vi "Drive Controller.vi"(8 "error in":errorcluster) -> ()   [LabVIEW 2015]
doc: "This VI executes continuously carrying out the current operation and responding to updates or new operations. It will often contain the timing or control code that is difficult to place directly in TeleOp. This VI generally opens all sensors and motors and isolates the rest of the robot code from knowing how the operations are carried out."
uses:
  Drive Setpoints.ctl
  Drive Operations.ctl
  <vilib>/Rock Robotics/WPI/CAN/TalonSRX/WPI_CANTalonSRX_APIControlMode.ctl
  <vilib>/Rock Robotics/WPI/DriverStation/WPI_DriverStationRobotMode2.ctl
  Drive Published Globals.vi
  Support Code/Team900-VIs/navX Library v2/navX Library v2.lvlib
panel:
  in  "Turn PID Gains (Drive for Distance)":T1 {"derivative time (Td, min)" format="%.3f"; "integral time (Ti, min)" format="%.3f"; "proportional gain (Kc)" format="%.3f"}
  in  "Max Speed":dbl format="%#_13g"
  out "Current\nCmd":string
  # "Tip: It may be helpful to observe inputs and sensor values.\nYou may also want to display tuning or debugging controls."
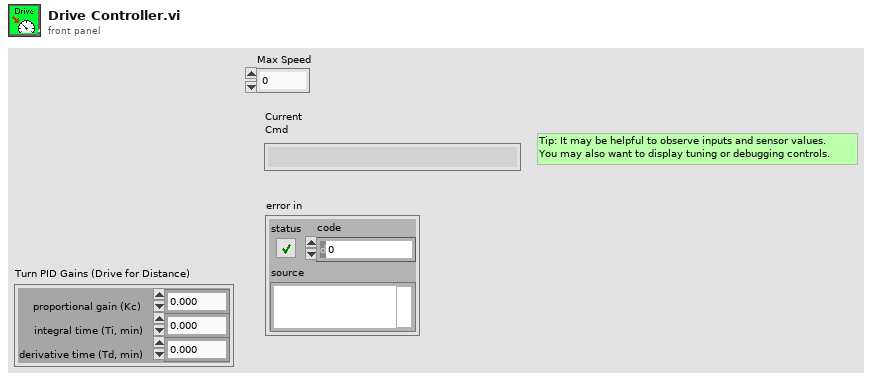
[diagram p1: front panel]
types:
  T1 = cluster{"proportional gain (Kc)":dbl, "integral time (Ti, min)":dbl, "derivative time (Td, min)":dbl}
  T2 = typedef "Drive Setpoints.ctl" = cluster{"Operation":T3, "Left Setpoint":dbl, "Duration":dbl, "Right Setpoint":dbl}
  T3 = typedef "Drive Operations.ctl" = enum16{"Reserve", "Read Current", "Immediate", "Turn to Angle", "Drive for Distance", "Drive for Time"}
  T4 = typedef "Command Status Info.ctl" = cluster{"Name":string, "Status":T5, "notifier out":T6}
  T5 = typedef "Completion Status.ctl" = enum16{"Successful", "Aborted", "Incomplete"}
  T6 = typedef "Completion Notifier.ctl" = refnum<notifier>
  T7 = cluster{"Default Command":T2, "Command Timing":cluster{"Start Time (ms)":u32, "Iterations":i32}, "Command Arguments":cluster{"Command Info":T4, "Description":string, "Default Command":T2, "notifier out":refnum<notifier>, "Subsystem Name":string}}
  T8 = typedef "navX Library v2.lvlib/Z900_navX_DeviceTypeDef.ctl" = cluster{"Interface":cluster{"Protocol":T9, "Update Rate (4Hz-60Hz)":u8, "navX Open TypeDef":variant}, "Notify Packet":refnum<notifier>, "Loop VI Refnum":refnum<vi>, "Ready to Close Occurrence Refnum":refnum<k4>}
  T9 = typedef "navX Library v2.lvlib/Z900_navX_ProtocolTypeDef.ctl" = enum16{"SERIAL", "I2C", "SPI"}
  T10 = typedef "WPI_RobotDriveDevRef.ctl" = cluster{"DevStatus":errorcluster, "Motors[]":T11[], "Square Inputs":bool, "Max Output":dbl}
  T11 = typedef "WPI_MotorControlDeviceRef.ctl" = cluster{"DeviceStatus":errorcluster, "Type":T12, "PWM":cluster{"PWM Channel":T13, "DeadBand":T14}, "CAN":cluster{"Device Number":u8, "Control Mode":T15, "Semaphore":T16, "Max Vout":dbl, "TalonSRX Control Mode":T17}, "Invert":bool}
  T12 = typedef "WPI_MotorControlType.ctl" = enum16{"PWM", "CAN", "CANTalonSRX"}
  T13 = typedef "FPGA_DIOPWMChannel.ctl" = enum8{"PWM 0", "PWM 1", "PWM 2", "PWM 3", "PWM 4", "PWM 5", "PWM 6", "PWM 7", "PWM 8", "PWM 9", "PWM MXP 0", "PWM MXP 1", "PWM MXP 2", "PWM MXP 3", "PWM MXP 4", "PWM MXP 5", "PWM MXP 6", "PWM MXP 7", "PWM MXP 8", "PWM MXP 9", "Invalid"}
  T14 = typedef "WPI_PWMDeadband.ctl" = cluster{"Name":string, "maxPositivePwm":i32, "minPositivePwm":i32, "centerPwm":i32, "maxNegativePwm":i32, "minNegativePwm":i32, "angularRange":u16}
  T15 = typedef "WPI_CANJaguar_ControlMode.ctl" = enum8{"Percent VBus", "Current", "Speed", "Position", "Voltage"}
  T16 = typedef "Semaphore RefNum" = refnum<k1>
  T17 = typedef "WPI_CANTalonSRX_APIControlMode.ctl" = enum8{"Percent VBus", "Speed", "Position", "Slave", "Unchanged / Invalid", "Voltage Compensation", "Current", "Motion Profile"}
  T18 = typedef "WPI_DriverStationRobotMode2.ctl" = enum16{"Autonomous Disabled", "Autonomous Enabled", "Teleop Disabled", "Teleop Enabled", "Disconnected", "Finish", "Test Disabled", "Test Enabled", "Emergency Stopped"}
  T19 = cluster{"Yaw":dbl, "Roll":dbl, "Pitch":dbl, "Heading":dbl, "Fused Heading":dbl}
  T20 = typedef "WPI_CANTalonSRX_GlobalStatus.ctl" = cluster{"Applied Throttle":dbl, "Module Enabled":bool, "CAN Error":errorcluster, "Closed Loop Error":dbl, "Forward Limit Switch Closed":bool, "Reverse Limit Switch Closed":bool, "Sensor Position":dbl, "Sensor Velocity":dbl, "Current":dbl, "Sticky Fault - Over Temp":bool, "Sticky Fault - Under Voltage":bool, "Sticky Fault - Forward Limit":bool, "Sticky Fault - Reverse Limit":bool, "Sticky Fault - Forward Soft Limit":bool, "Sticky Fault - Reverse Soft Limit":bool, "Brake is Enabled":bool, "Encoder Position":dbl, "Encoder Velocity":dbl, "Encoder Index Count":dbl, "Encoder A Pin State":bool, "Encoder B Pin State":bool, "Encoder Index Pin State":bool, "Analog In":dbl, "Analog In Velocity":dbl, "Temperature (C)":dbl, "Battery Voltage":dbl, "Control 5 Is Supported":bool, "Current Profile Slot Select":dbl, "Pos Div 8":bool, "Vel Div 4":bool, "Pulse Width Position":i32, "Pulse Width Velocity":i32, "Pulse Width Rise To Rise (us)":i32, "Pulse Width Rise To Fall (us)":i32, "Mot Prof Active Is Under Run":bool, "Mot Prof Active Has Under Run":bool, "Mot Prof Active Is Last":bool, "Mot Prof Active Velocity Only":bool, "Mot Prof Active Is Valid":bool, "Mot Prof Buffer Is Full":bool, "Mot Prof Active Profile Slot Select":i32, "Mot Prof NextID":i32, "Mot Prof Count":i32, "Mot Prof Active Velocity":dbl, "Mot Prof Active Position":dbl, "Mot Prof Output Enable":i32}
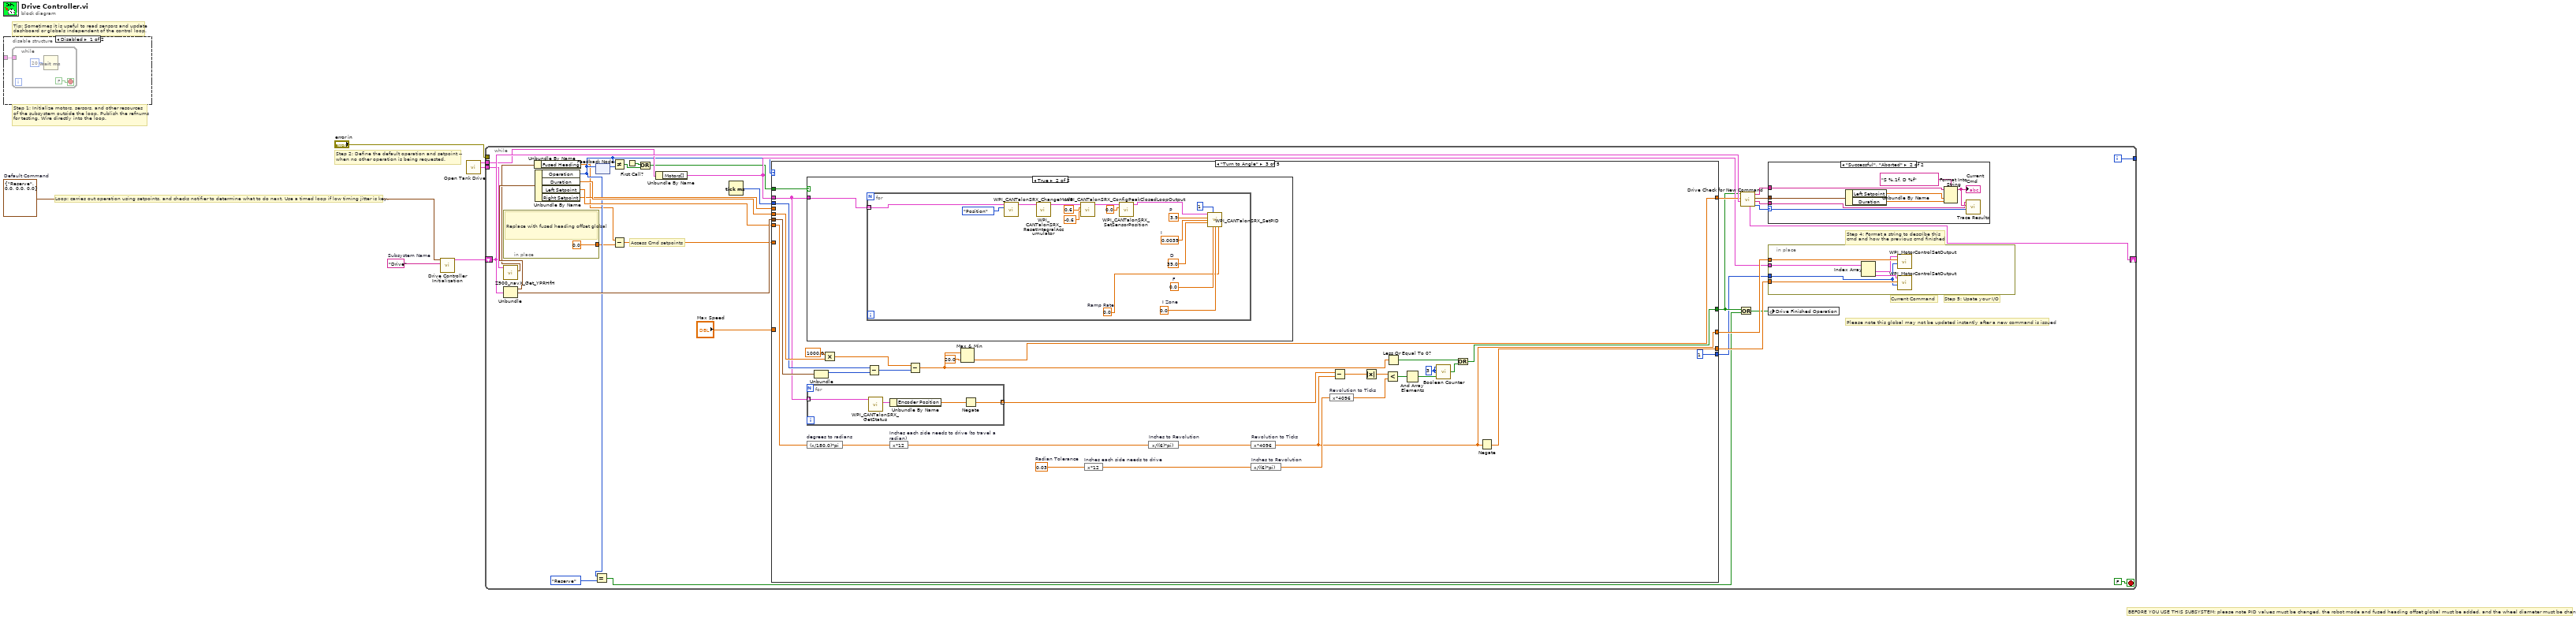
[diagram p0: block diagram]
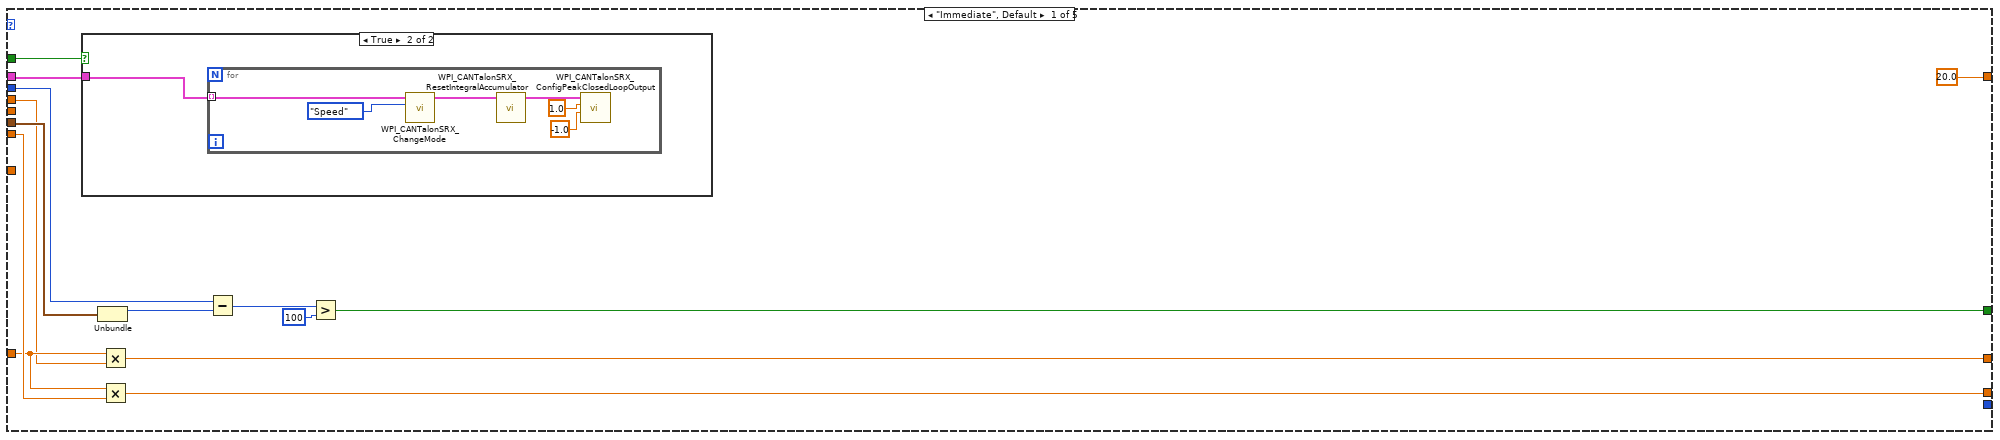
[diagram p4: hidden frame]
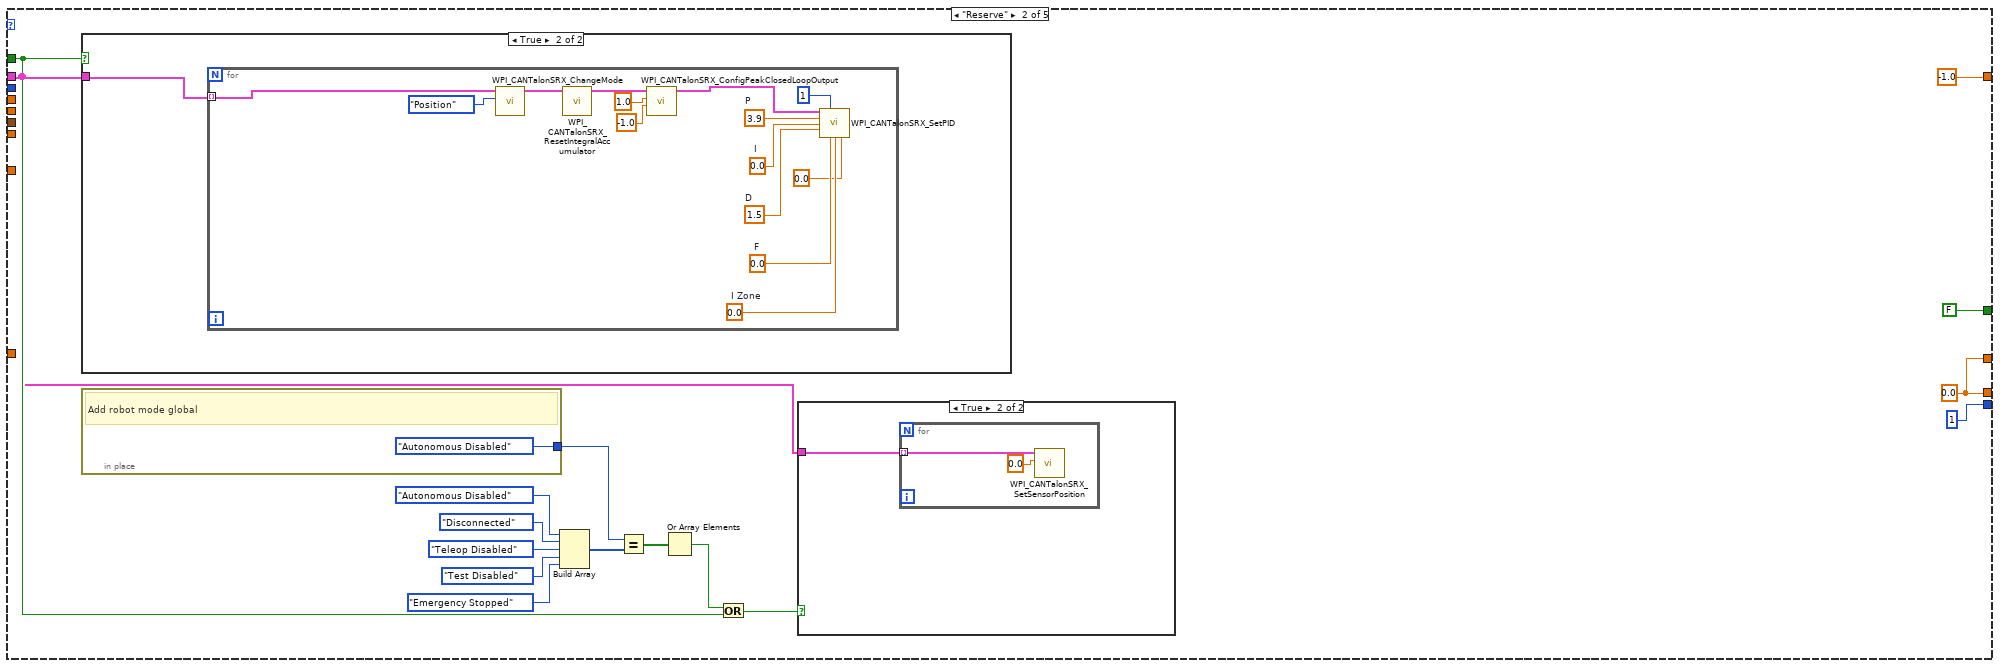
[diagram p6: hidden frame]
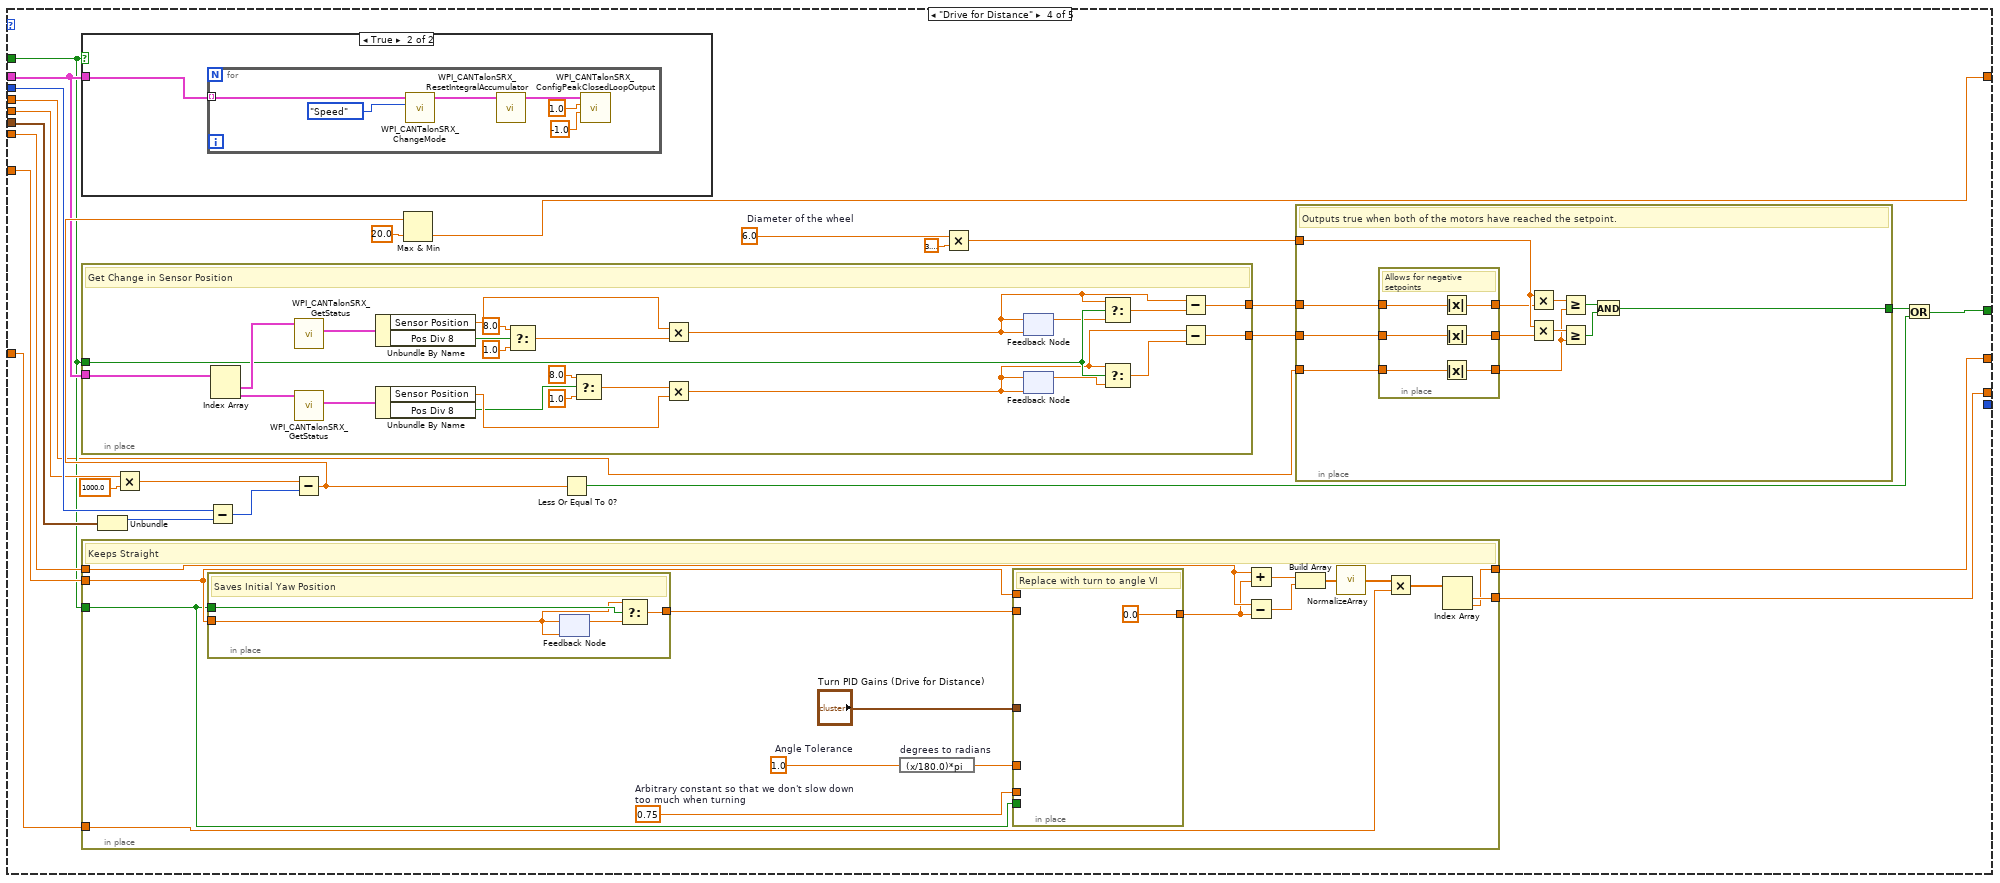
[diagram p10: hidden frame]
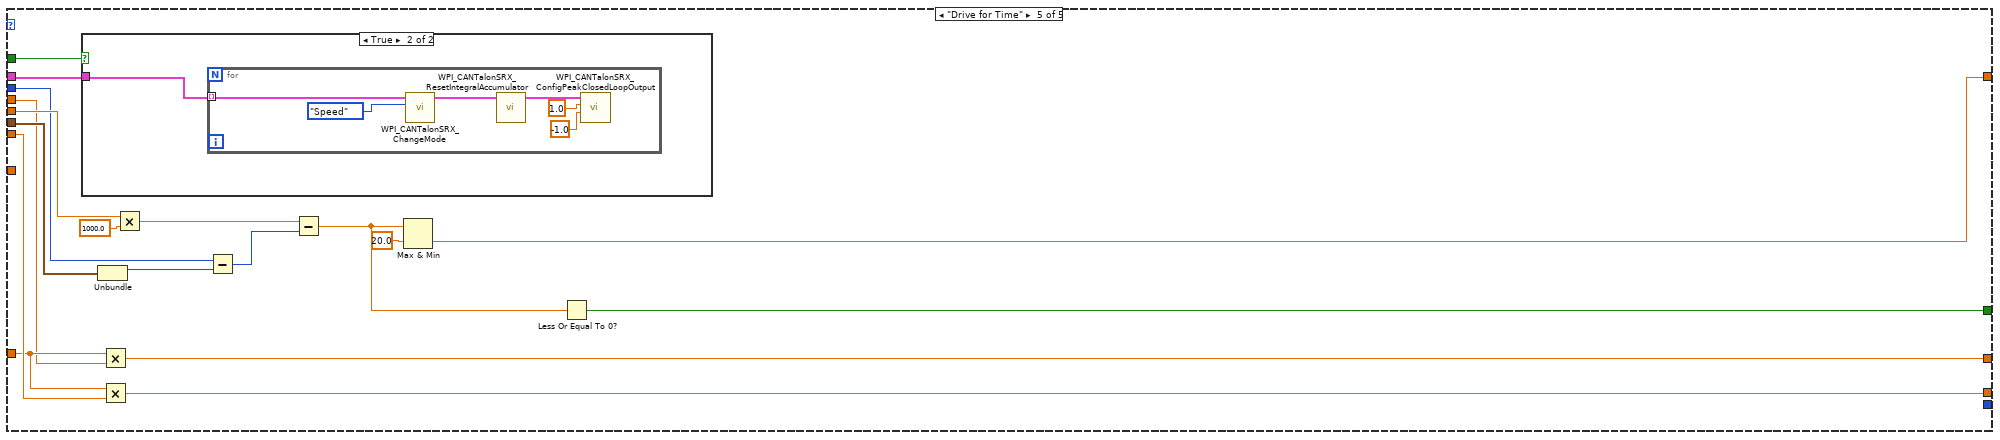
[diagram p12: hidden frame]
diagram:
  w3 = T2 {"Operation"=enum."Reserve", "Left Setpoint"=0.0, "Duration"=0.0, "Right Setpoint"=0.0}  # Default Command
  w4 = "Drive"  # Subsystem Name
  # "BEFORE YOU USE THIS SUBSYSTEM: please note PID values must be changed, the robot mode and fused heading offset global must be added, and the wheel diameter must be changed"
  # "Tip: Sometimes it is useful to read sensors and update\ndashboard or globals independent of the control loop."
  # "Step 2: Define the default operation and setpoint --\nwhen no other operation is being requested."
  # "Step 1: Initialize motors, sersors, and other resources\nof the subsystem outside the loop. Publish the refnums\nfor testing. Wire directly into the loop."
  # "Loop: carries out operation using setpoints, and checks notifier to determine what to do next. Use a timed loop if low timing jitter is key."
  n1 = disable-structure shown="Disabled" {
    disable-tunnel: _ -> [w7 _]
    frame Disabled {
      n2 = while {
        tunnel: w7 -> [_]
        stop <- FALSE stop-if-true
        n3 = Wait (ms)(milliseconds to wait=u32 20) -> ()  [unwired: 1 out]
      }
    }
    frame Enabled {
    }
  }
  n4 = call "Drive Controller Initialization.vi"("Subsystem Name"=w4, "Default Command"=w3) -> ("Command Info"=w5:T7)  [unwired: 9 in]
  n5 = call "Open Tank Drive.vi"() -> ("navX Device"=w1:T8, "RobotDriveDevRef"=w2:T10)  [unwired: 1 out]
  n6 = while {
    shift-right: [w36] -> _
    shift-left: w5 -> [w37]
    tunnel: [w43] -> _
    tunnel: "error in" -> [_]
    tunnel: w2 -> [w26]
    tunnel: w1 -> [w15]
    i -> [w43]
    stop <- FALSE stop-if-true
    # "Please note this global may not be updated instantly after a new command is issued"
    # "Step 5: Upate your I/O"
    # "Step 4: Format a string to describe this\ncmd and how the previous cmd finished"
    # "Current Command"
    # "Access Cmd setpoints"
    n7 = in-place {
      in-place-border: [0.0 ("y")] -> w11
      # "Replace with fused heading offset global"
    }
    n8 = call "Z900_navX_Get_YPRHfH.vi"("navX Device"=w15) -> ("YRPHfH"=w13:T19)  [unwired: 7 in, 3 out]
    n9 = Unbundle(w37) -> ("Default Command"=w42:T2, "Command Timing"=w39:cluster{"Start Time (ms)":u32, "Iterations":i32})  [unwired: 1 out]
    n10 = Unbundle By Name(w13) -> ("Fused Heading"=w12:dbl)
    n11 = Unbundle By Name(w42) -> ("Operation"=w19:T3, "Duration"=w41:dbl, "Left Setpoint"=w38:dbl, "Right Setpoint"=w29:dbl)
    n12 = Equal?(x=w19, y=Drive_Operations."Reserve") -> (x = y?=w17:bool)
    n13 = feedback-in #1(w19) -> ()
    n14 = feedback #1() -> (w25:T3)  [unwired: 1 in]
    n15 = Not Equal?(x=w19, y=w25) -> (x != y?=w24:bool)
    n16 = Subtract(x=w12, y=w11) -> (x-y=w10:dbl)
    n17 = First Call?() -> (First Call?: T/F=w21:bool)
    n18 = Or(x=w21, y=w24) -> (x .or. y?=w22:bool)
    n19 = Unbundle By Name(w26) -> ("Motors[]"=w23:T11[])
    n20 = Tick Count (ms)() -> (millisecond timer value=w40:u32)
    n21 = case shown="\"Turn to Angle\"" w19 {
      tunnel: [20.0 -1.0 w140 w188 w278] -> w35
      tunnel: [w67 FALSE ("ignore previous (F)") w120 w170 w279] -> w20
      tunnel: w39 -> [w69 _ w141 w189 w275]
      tunnel: w41 -> [_ _ w143 w180 w277]
      tunnel: w40 -> [w68 _ w142 w190 w276]
      tunnel: w38 -> [w66 _ w127 w186 w274]
      tunnel: "Max Speed" -> [w65 _ _ w184 w270]
      tunnel: w29 -> [w64 _ _ w171 w269]
      tunnel: [w63 w94 w126 w183 w273] -> w28
      tunnel: [w62 w94 w125 w182 w268] -> w27
      tunnel: w22 -> [w61 w84 w123 w173 w271]
      tunnel: w23 -> [w60 w82 w124 w174 w272]
      tunnel: w10 -> [_ _ _ w185 _]
      tunnel: [_ 1 1 _ _] -> w14
      frame "Immediate", Default {
        n22 = case shown="True" w61 {
          tunnel: w60 -> [_ w74]
          frame False {
          }
          frame True {
            n23 = for {
              tunnel: w74 -> [w80] mode=indexing
              n24 = call <vilib>:"WPI_CANTalonSRX_ChangeMode.vi"("Control Mode"=WPI_CANTalonSRX_APIControlMode."Speed", "CAN Talon SRX Ref"=w80) -> ("CAN Talon SRX Ref"=w78:T11)  [unwired: 8 in, 1 out]
              n25 = call <vilib>:"WPI_CANTalonSRX_ResetIntegralAccumulator.vi"("CAN Talon SRX Ref"=w78) -> ("CAN Talon SRX Ref"=w77:T11)  [unwired: 9 in, 1 out]
              n26 = call <vilib>:"WPI_CANTalonSRX_ConfigPeakClosedLoopOutput.vi"("Reverse Peak Output"=-1.0, "Forward Peak Output"=1.0, "CAN Talon SRX Ref"=w77) -> ()  [unwired: 7 in, 2 out]
            }
          }
        }
        n27 = Unbundle(w69) -> ("Start Time (ms)"=w72:u32)  [unwired: 1 out]
        n28 = Multiply(x=w65, y=w64) -> (x*y=w62:dbl)
        n29 = Multiply(x=w65, y=w66) -> (x*y=w63:dbl)
        n30 = Subtract(x=w68, y=w72) -> (x-y=w71:u32)
        n31 = Greater?(x=w71, y=u8 100 ("Left Motor")) -> (0:w67:bool)
      }
      frame "Reserve" {
        w94 = 0.0
        n32 = case shown="True" w84 {
          tunnel: w82 -> [_ w101]
          frame False {
          }
          frame True {
            n33 = for {
              tunnel: w101 -> [w115] mode=indexing
              w106 = 0.0  # I Zone
              w104 = 0.0  # F
              w103 = 1.5  # D
              w107 = 0.0  # I
              w108 = 3.9  # P
              n34 = call <vilib>:"WPI_CANTalonSRX_ChangeMode.vi"("Control Mode"=WPI_CANTalonSRX_APIControlMode."Position", "CAN Talon SRX Ref"=w115) -> ("CAN Talon SRX Ref"=w110:T11)  [unwired: 8 in, 1 out]
              n35 = call <vilib>:"WPI_CANTalonSRX_ResetIntegralAccumulator.vi"("CAN Talon SRX Ref"=w110) -> ("CAN Talon SRX Ref"=w113:T11)  [unwired: 9 in, 1 out]
              n36 = call <vilib>:"WPI_CANTalonSRX_ConfigPeakClosedLoopOutput.vi"("Reverse Peak Output"=-1.0, "Forward Peak Output"=1.0, "CAN Talon SRX Ref"=w113) -> ("CAN Talon SRX Ref"=w109:T11)  [unwired: 7 in, 1 out]
              n37 = call <vilib>:"WPI_CANTalonSRX_SetPID.vi"("CAN Talon SRX Ref"=w109, "Parameter Slot"=u8 1, "P"=w108, "I"=w107, "D"=w103, "F"=w104, "I Zone"=w106, "Ramp Rate"=0.0) -> ()  [unwired: 6 in, 2 out]
            }
          }
        }
        n38 = in-place {
          in-place-border: [WPI_DriverStationRobotMode2."Autonomous Disabled" ("y")] -> w86
          # "Add robot mode global"
        }
        n39 = Build Array(WPI_DriverStationRobotMode2."Autonomous Disabled" ("y"), WPI_DriverStationRobotMode2."Disconnected" ("y"), WPI_DriverStationRobotMode2."Teleop Disabled" ("y"), WPI_DriverStationRobotMode2."Test Disabled" ("y"), WPI_DriverStationRobotMode2."Emergency Stopped" ("y")) -> (w88:T18[])
        n40 = Equal?(x=w86, y=w88) -> (x = y?=w87:bool[])
        n41 = Or Array Elements(Boolean array=w87) -> (logical OR=w85:bool)
        n42 = Or(x=w85, y=w84) -> (x .or. y?=w83:bool)
        n43 = case shown="True" w83 {
          tunnel: w82 -> [_ w97]
          frame False {
          }
          frame True {
            n44 = for {
              tunnel: w97 -> [w98] mode=indexing
              n45 = call <vilib>:"WPI_CANTalonSRX_SetSensorPosition.vi"("New Sensor Position"=0.0, "CAN Talon SRX Ref"=w98) -> ()  [unwired: 8 in, 2 out]
            }
          }
        }
      }
      frame "Turn to Angle" {
        w121 = 3 ("Array Size")
        w129 = 0.03  # Radian Tolerance
        n46 = case shown="True" w123 {
          tunnel: w124 -> [_ w152]
          frame False {
          }
          frame True {
            n47 = for {
              tunnel: w152 -> [w168] mode=indexing
              w154 = 0.0  # Ramp Rate
              w158 = 0.0  # I Zone
              w156 = 0.0  # F
              w155 = 39.0  # D
              w159 = 0.0039  # I
              w160 = 3.9  # P
              n48 = call <vilib>:"WPI_CANTalonSRX_ChangeMode.vi"("Control Mode"=WPI_CANTalonSRX_APIControlMode."Position", "CAN Talon SRX Ref"=w168) -> ("CAN Talon SRX Ref"=w166:T11)  [unwired: 8 in, 1 out]
              n49 = call <vilib>:"WPI_CANTalonSRX_ResetIntegralAccumulator.vi"("CAN Talon SRX Ref"=w166) -> ("CAN Talon SRX Ref"=w165:T11)  [unwired: 9 in, 1 out]
              n50 = call <vilib>:"WPI_CANTalonSRX_ConfigPeakClosedLoopOutput.vi"("Reverse Peak Output"=-0.6, "Forward Peak Output"=0.6, "CAN Talon SRX Ref"=w165) -> ("CAN Talon SRX Ref"=w162:T11)  [unwired: 7 in, 1 out]
              n51 = call <vilib>:"WPI_CANTalonSRX_SetSensorPosition.vi"("New Sensor Position"=0.0, "CAN Talon SRX Ref"=w162) -> ("CAN Talon SRX Ref"=w153:T11)  [unwired: 8 in, 1 out]
              n52 = call <vilib>:"WPI_CANTalonSRX_SetPID.vi"("CAN Talon SRX Ref"=w153, "Parameter Slot"=u8 1, "P"=w160, "I"=w159, "D"=w155, "F"=w156, "I Zone"=w158, "Ramp Rate"=w154) -> ()  [unwired: 6 in, 2 out]
            }
          }
        }
        n53 = for {
          tunnel: w124 -> [w151] mode=indexing
          tunnel: [w148] -> w134 mode=indexing
          n54 = call <vilib>:"WPI_CANTalonSRX_GetStatus.vi"("CAN Talon SRX Ref"=w151) -> ("Talon SRX Status"=w150:T20)  [unwired: 8 in, 2 out]
          n55 = Unbundle By Name(w150) -> ("Encoder Position"=w149:dbl)
          n56 = Negate(x=w149) -> (-x=w148:dbl)
        }
        n57 = expression code="(x/180.0)*pi" "degrees to radians"(w127) -> (w138:dbl)
        n58 = Unbundle(w141) -> ("Start Time (ms)"=w145:u32)  [unwired: 1 out]
        n59 = Multiply(x=1000.0, y=w143) -> (x*y=w118:dbl)
        n60 = Subtract(x=w142, y=w145) -> (x-y=w146:u32)
        n61 = expression code="x*12" "Inches each side needs to drive (to travel a radian)"(w138) -> (w137:dbl)
        n62 = Subtract(x=w118, y=w146) -> (x-y=w147:dbl)
        n63 = Max & Min(x=w147, y=20.0) -> (min(x,y)=w140:dbl)  [unwired: 1 out]
        n64 = expression code="x*12" "Inches each side needs to drive"(w129) -> (w131:dbl)
        n65 = expression code="x/((6)*pi)" "Inches to Revolution"(w137) -> (w136:dbl)
        n66 = expression code="x*4096" "Revolution to Ticks"(w136) -> (w125:dbl)
        n67 = expression code="x/((6)*pi)" "Inches to Revolution"(w131) -> (w130:dbl)
        n68 = expression code="x*4096" "Revolution to Ticks"(w130) -> (w128:dbl)
        n69 = Subtract(x=w134, y=w125) -> (x-y=w133:dbl[])
        n70 = Absolute Value(x=w133) -> (abs(x)=w132:dbl[])
        n71 = Less?(x=w132, y=w128) -> (x < y?=w135:bool[])
        n72 = Less Or Equal To 0?(x=w147) -> (x <= 0?=w139:bool)
        n73 = And Array Elements(Boolean array=w135) -> (logical AND=w122:bool)
        n74 = call "Boolean Counter.vi"("Input Boolean"=w122, "Min of array which must be true"=w121, "Array Size"=w121) -> ("Output Boolean"=w119:bool)
        n75 = Or(x=w139, y=w119) -> (x .or. y?=w120:bool)
        n76 = Negate(x=w125) -> (-x=w126:dbl)
      }
      frame "Drive for Distance" {
        w177 = 6.0  # Diameter of the wheel
        n77 = case shown="True" w173 {
          tunnel: w174 -> [_ w237]
          frame False {
          }
          frame True {
            n78 = for {
              tunnel: w237 -> [w243] mode=indexing
              n79 = call <vilib>:"WPI_CANTalonSRX_ChangeMode.vi"("Control Mode"=WPI_CANTalonSRX_APIControlMode."Speed", "CAN Talon SRX Ref"=w243) -> ("CAN Talon SRX Ref"=w238:T11)  [unwired: 8 in, 1 out]
              n80 = call <vilib>:"WPI_CANTalonSRX_ResetIntegralAccumulator.vi"("CAN Talon SRX Ref"=w238) -> ("CAN Talon SRX Ref"=w241:T11)  [unwired: 9 in, 1 out]
              n81 = call <vilib>:"WPI_CANTalonSRX_ConfigPeakClosedLoopOutput.vi"("Reverse Peak Output"=-1.0, "Forward Peak Output"=1.0, "CAN Talon SRX Ref"=w241) -> ()  [unwired: 7 in, 2 out]
            }
          }
        }
        n82 = in-place {
          in-place-border: w173 -> [w214]
          in-place-border: [w209] -> w176
          in-place-border: [w208] -> w175
          in-place-border: w174 -> [w195]
          # "Get Change in Sensor Position"
          n83 = Index Array(array=w195) -> (element #1=w218:T11, element #2=w217:T11)  [unwired: 2 in]
          n84 = call <vilib>:"WPI_CANTalonSRX_GetStatus.vi"("CAN Talon SRX Ref"=w218) -> ("Talon SRX Status"=w216:T20)  [unwired: 8 in, 2 out]
          n85 = call <vilib>:"WPI_CANTalonSRX_GetStatus.vi"("CAN Talon SRX Ref"=w217) -> ("Talon SRX Status"=w215:T20)  [unwired: 8 in, 2 out]
          n86 = Unbundle By Name(w216) -> ("Sensor Position"=w211:dbl, "Pos Div 8"=w198:bool)
          n87 = Unbundle By Name(w215) -> ("Sensor Position"=w210:dbl, "Pos Div 8"=w207:bool)
          n88 = Select(t=8.0, s=w198, f=1.0) -> (s? t:f=w199:dbl)
          n89 = Select(t=8.0, s=w207, f=1.0) -> (s? t:f=w203:dbl)
          n90 = Multiply(x=w211, y=w199) -> (x*y=w200:dbl)
          n91 = Multiply(x=w203, y=w210) -> (x*y=w204:dbl)
          n92 = feedback #2(w200) -> (w196:dbl)
          n93 = feedback-in #2(w200) -> ()
          n94 = feedback #3(w204) -> (w197:dbl)
          n95 = feedback-in #3(w204) -> ()
          n96 = Select(t=w200, s=w214, f=w196) -> (s? t:f=w213:dbl)
          n97 = Select(t=w204, s=w214, f=w197) -> (s? t:f=w212:dbl)
          n98 = Subtract(x=w200, y=w213) -> (x-y=w209:dbl)
          n99 = Subtract(x=w204, y=w212) -> (x-y=w208:dbl)
        }
        n100 = in-place {
          in-place-border: w173 -> [w246]
          in-place-border: w185 -> [w252]
          in-place-border: [w254] -> w183
          in-place-border: w186 -> [w251]
          in-place-border: [w253] -> w182
          in-place-border: w184 -> [w244]
          w259 = 1.0  # Angle Tolerance
          w260 = 0.75  # Arbitrary constant so that we don't slow down too much when turning
          # "Keeps Straight"
          n101 = in-place {
            in-place-border: w252 -> [w264]
            in-place-border: w246 -> [w265]
            in-place-border: [w262] -> w249
            # "Saves Initial Yaw Position"
            n102 = feedback #4(w264) -> (w263:dbl)
            n103 = feedback-in #4(w264) -> ()
            n104 = Select(t=w264, s=w265, f=w263) -> (s? t:f=w262:dbl)
          }
          n105 = expression code="(x/180.0)*pi" "degrees to radians"(w259) -> (w248:dbl)
          n106 = in-place {
            in-place-border: w260 -> [_]
            in-place-border: w252 -> [_]
            in-place-border: "Turn PID Gains (Drive for Distance)" -> [_]
            in-place-border: w249 -> [_]
            in-place-border: w248 -> [_]
            in-place-border: [0.0 ("Turn Speed (subtract from the left motor output)")] -> w247
            in-place-border: w246 -> [_]
            # "Replace with turn to angle VI"
          }
          n107 = Add(x=w251, y=w247) -> (x+y=w255:dbl)
          n108 = Subtract(x=w251, y=w247) -> (x-y=w258:dbl)
          n109 = Build Array(w255, w258) -> (w257:dbl[])
          n110 = call "NormalizeArray.vi"("array"=w257) -> ("normalized array"=w256:dbl[])
          n111 = Multiply(x=w256, y=w244) -> (x*y=w245:dbl[])
          n112 = Index Array(array=w245) -> (element #1=w254:dbl, element #2=w253:dbl)  [unwired: 2 in]
        }
        n113 = Unbundle(w189) -> ("Start Time (ms)"=w192:u32)  [unwired: 1 out]
        n114 = Multiply(x=w180, y=1000.0) -> (x*y=w179:dbl)
        n115 = Subtract(x=w190, y=w192) -> (x-y=w193:u32)
        n116 = Subtract(x=w179, y=w193) -> (x-y=w194:dbl)
        n117 = Max & Min(x=w194, y=20.0) -> (min(x,y)=w188:dbl)  [unwired: 1 out]
        n118 = Less Or Equal To 0?(x=w194) -> (x <= 0?=w187:bool)
        n119 = Multiply(x=w177, y=3.141592653589793) -> (x*y=w172:dbl)
        n120 = in-place {
          in-place-border: w171 -> [w223]
          in-place-border: w172 -> [w226]
          in-place-border: w176 -> [w221]
          in-place-border: w175 -> [w220]
          in-place-border: [w219] -> w169
          # "Outputs true when both of the motors have reached the setpoint."
          n121 = in-place {
            in-place-border: w221 -> [w236]
            in-place-border: w220 -> [w235]
            in-place-border: [w234] -> w225
            in-place-border: [w233] -> w224
            in-place-border: w223 -> [w232]
            in-place-border: [w231] -> w222
            # "Allows for negative setpoints"
            n122 = Absolute Value(x=w236) -> (abs(x)=w234:dbl)
            n123 = Absolute Value(x=w235) -> (abs(x)=w233:dbl)
            n124 = Absolute Value(x=w232) -> (abs(x)=w231:dbl)
          }
          n125 = Multiply(x=w226, y=w225) -> (x*y=w229:dbl)
          n126 = Multiply(x=w226, y=w224) -> (x*y=w230:dbl)
          n127 = Greater Or Equal?(x=w229, y=w222) -> (x >= y?=w228:bool)
          n128 = Greater Or Equal?(x=w230, y=w222) -> (x >= y?=w227:bool)
          n129 = And(x=w228, y=w227) -> (x .and. y?=w219:bool)
        }
        n130 = Or(x=w169, y=w187) -> (x .or. y?=w170:bool)
      }
      frame "Drive for Time" {
        n131 = case shown="True" w271 {
          tunnel: w272 -> [_ w284]
          frame False {
          }
          frame True {
            n132 = for {
              tunnel: w284 -> [w290] mode=indexing
              n133 = call <vilib>:"WPI_CANTalonSRX_ChangeMode.vi"("Control Mode"=WPI_CANTalonSRX_APIControlMode."Speed", "CAN Talon SRX Ref"=w290) -> ("CAN Talon SRX Ref"=w285:T11)  [unwired: 8 in, 1 out]
              n134 = call <vilib>:"WPI_CANTalonSRX_ResetIntegralAccumulator.vi"("CAN Talon SRX Ref"=w285) -> ("CAN Talon SRX Ref"=w288:T11)  [unwired: 9 in, 1 out]
              n135 = call <vilib>:"WPI_CANTalonSRX_ConfigPeakClosedLoopOutput.vi"("Reverse Peak Output"=-1.0, "Forward Peak Output"=1.0, "CAN Talon SRX Ref"=w288) -> ()  [unwired: 7 in, 2 out]
            }
          }
        }
        n136 = Unbundle(w275) -> ("Start Time (ms)"=w281:u32)  [unwired: 1 out]
        n137 = Multiply(x=w270, y=w269) -> (x*y=w268:dbl)
        n138 = Multiply(x=w270, y=w274) -> (x*y=w273:dbl)
        n139 = Multiply(x=w277, y=1000.0) -> (x*y=w267:dbl)
        n140 = Subtract(x=w276, y=w281) -> (x-y=w282:u32)
        n141 = Subtract(x=w267, y=w282) -> (x-y=w283:dbl)
        n142 = Max & Min(x=w283, y=20.0) -> (min(x,y)=w278:dbl)  [unwired: 1 out]
        n143 = Less Or Equal To 0?(x=w283) -> (x <= 0?=w279:bool)
      }
    }
    n144 = Or(x=w20, y=w17) -> (x .or. y?=w16:bool)
    n145 = call "Drive Check for New Command.vi"("Current Command"=w37, "Wait time (ms)"=w35, "Finished?"=w20) -> ("Completion"=w31:T5, "Subsystem Name"=w32:string, "Current Command"=w33:T2, "Initial Trace String"=w34:string, "NextCommand"=w36:T7)  [unwired: 4 in]
    n146 = case shown="\"Successful\", \"Aborted\"" w31 {
      selector: w31 -> [_ w59]
      tunnel: w34 -> [_ w55]
      tunnel: w33 -> [_ w56]
      tunnel: w32 -> [_ w52]
      frame "Incomplete", Default {
        # "Continuing current command"
      }
      frame "Successful", "Aborted" {
        # "Report and setup for next command"
        n147 = Unbundle By Name(w56) -> ("Left Setpoint"=w58:dbl, "Duration"=w53:dbl)
        n148 = Format Into String(format string="S %.1f, D %f", initial string=w55, w58, w53) -> (resulting string=w54:string)  [unwired: 1 in, 1 out]
        "Current\nCmd" <- w54
        n149 = call <vilib>:"Trace Results.vi"("Status of previous command"=w59, "Description"=w54, "Subsystem"=w52) -> ()  [unwired: 9 in]
      }
    }
    n150 = in-place {
      in-place-border: w28 -> [w51]
      in-place-border: w27 -> [w50]
      in-place-border: w23 -> [w49]
      in-place-border: w14 -> [w46]
      n151 = Index Array(array=w49) -> (element #1=w47:T11, element #2=w48:T11)  [unwired: 2 in]
      n152 = call <vilib>:"WPI_MotorControlSetOutput.vi"("Sync Group / Parameter Slot"=w46, "Output"=w50, "MotorControlDevRef"=w47) -> ()  [unwired: 6 in, 3 out]
      n153 = call <vilib>:"WPI_MotorControlSetOutput.vi"("Sync Group / Parameter Slot"=w46, "Output"=w51, "MotorControlDevRef"=w48) -> ()  [unwired: 6 in, 3 out]
    }
    n154 = global write "Drive Published Globals.vi" "Drive Finished Operation"(w16) -> ()
  }
